vi "GSM_MASK_FREQ.vi"(4 "RO":bool, 6 "REF(MHz)":dbl, 8 "error in":errorcluster {"code" format="%.0x"}, 11 "Session In":refnum<visa-resource-name>="TCPIP0::K-N90X0A-00005.local::hislip0::INSTR") -> (0 "error out":errorcluster {"code" format="%.0x"}, 3 "Session Out":refnum<visa-resource-name>, 5 "RefFreq(MHz)":dbl)   [LabVIEW 2018]
panel:
  in  "Timeout":u32=3000
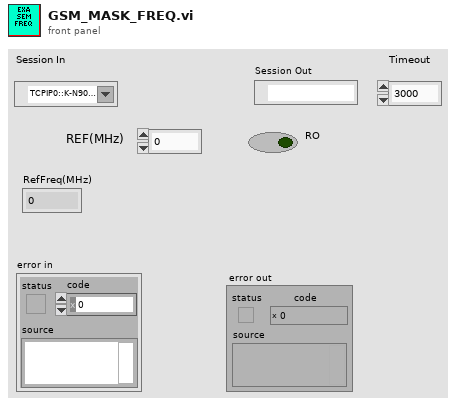
[diagram p1: front panel]
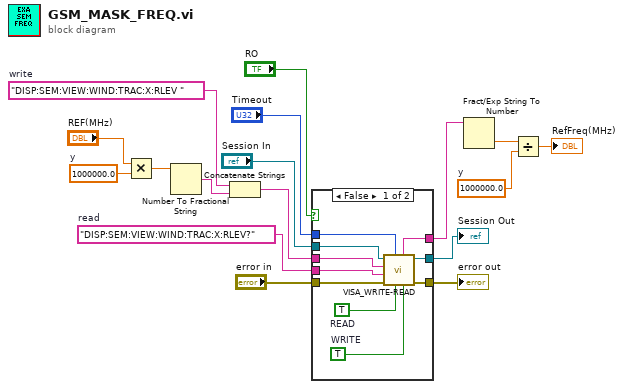
[diagram p0: block diagram]
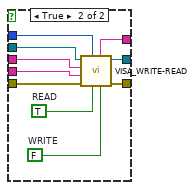
[diagram p2: hidden frame]
diagram:
  w5 = 1000000.0  # y
  w13 = "DISP:SEM:VIEW:WIND:TRAC:X:RLEV?"  # read
  w15 = "DISP:SEM:VIEW:WIND:TRAC:X:RLEV "  # write
  w7 = 1000000.0  # y
  n1 = Multiply(x="REF(MHz)", y=w5) -> (x*y=w4:dbl)
  n2 = Number To Fractional String(number=w4) -> (F-format string=w3:string)  [unwired: 3 in]
  n3 = Concatenate Strings(w15, w3) -> (w14:string)
  n4 = case shown="False" "RO" {
    tunnel: "error in" -> [w27 w37]
    tunnel: [w26 w36] -> w16
    tunnel: w14 -> [w25 w35]
    tunnel: w13 -> [w24 w34]
    tunnel: "Session In" -> [w23 w33]
    tunnel: [w22 w32] -> w11
    tunnel: [w21 w31] -> w10
    tunnel: "Timeout" -> [w20 w30]
    frame False {
      w18 = TRUE  # WRITE
      w19 = TRUE  # READ
      n5 = call "VISA_WRITE-READ.vi"("WRITE"=w18, "READ"=w19, "Timeout"=w20, "error in"=w27, "Rcmd"=w24, "Wcmd"=w25, "Session In"=w23) -> ("error out"=w26:errorcluster, "Session Out"=w22:refnum<visa-resource-name>, "Out"=w21:string)  [unwired: 2 in]
    }
    frame True {
      w28 = FALSE  # WRITE
      w29 = TRUE  # READ
      n6 = call "VISA_WRITE-READ.vi"("WRITE"=w28, "READ"=w29, "Timeout"=w30, "error in"=w37, "Rcmd"=w34, "Wcmd"=w35, "Session In"=w33) -> ("error out"=w36:errorcluster, "Session Out"=w32:refnum<visa-resource-name>, "Out"=w31:string)  [unwired: 2 in]
    }
  }
  "error out" <- w16
  "Session Out" <- w11
  n7 = Fract/Exp String To Number(string=w10) -> (number=w8:dbl)  [unwired: 3 in, 1 out]
  n8 = Divide(x=w8, y=w7) -> (x/y=→"RefFreq(MHz)":dbl)
